vi "increment filename.vi"(1 "path":path) -> (0 "modified path":path)   [LabVIEW 2016]
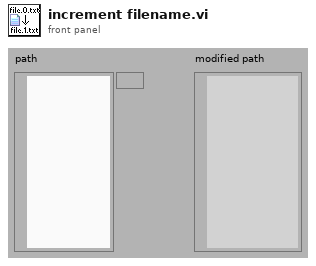
[diagram p1: front panel]
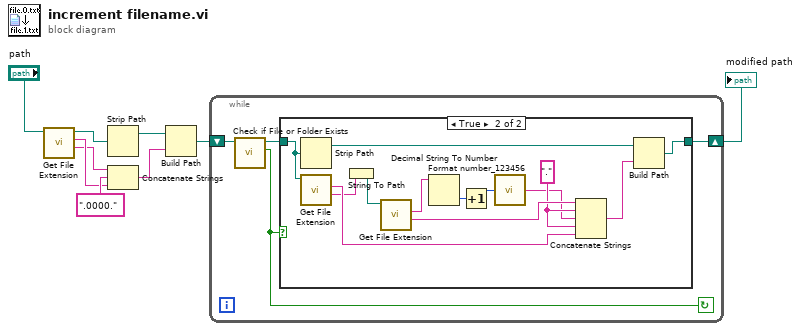
[diagram p0: block diagram]
diagram:
  n1 = call <vilib>:"Get File Extension.vi"("file"="path") -> ("filename without extension"=w6:string, "lowercase file extension"=w7:string, "dup file"=w3:path)  [unwired: 1 in, 7 out]
  n2 = Strip Path(path=w3) -> (stripped path=w2:path)  [unwired: 1 out]
  n3 = Concatenate Strings(w6, ".0000.", w7) -> (w1:string)
  n4 = Build Path(base path=w2, name or relative path=w1) -> (appended path=w5:path)
  n5 = while {
    shift-right: [w11] -> w9
    shift-left: w5 -> [w12]
    stop <- w10 continue-if-true
    n6 = call <vilib>:"Check if File or Folder Exists.vi"("path"=w12) -> ("file or folder exists?"=w10:bool, "dup path"=w13:path)  [unwired: 1 in, 8 out]
    n7 = case shown="True" w10 {
      tunnel: w13 -> [w14 w27]
      tunnel: [w14 w25] -> w11
      frame False {
      }
      frame True {
        w17 = "." ("regular expression")
        n8 = Strip Path(path=w27) -> (stripped path=w26:path)  [unwired: 1 out]
        n9 = call <vilib>:"Get File Extension.vi"("file"=w27) -> ("filename without extension"=w21:string, "lowercase file extension"=w23:string)  [unwired: 1 in, 8 out]
        n10 = String To Path(string=w21) -> (path=w20:path)
        n11 = call <vilib>:"Get File Extension.vi"("file"=w20) -> ("filename without extension"=w18:string, "lowercase file extension"=w19:string)  [unwired: 1 in, 8 out]
        n12 = Decimal String To Number(string=w19) -> (number=w24:i32)  [unwired: 1 in, 2 out]
        n13 = Increment(x=w24) -> (x+1=w15:i32)
        n14 = call <userlib>:"Format number_123456.vi"("number"=w15) -> ("String"=w16:string)
        n15 = Concatenate Strings(w18, w17, w16, w17, w23) -> (w22:string)
        n16 = Build Path(base path=w26, name or relative path=w22) -> (appended path=w25:path)
      }
    }
  }
  "modified path" <- w9
